vi "Prober_ProbeTouchdown.vi"(8 "error in (no error)":errorcluster, 11 "AlessiRel6100 in":refnum<class "AlessiRel6100.lvclass">) -> (0 "error out":errorcluster, 1 "previous Z [µm]":i32, 2 "Z [µm]":i32, 3 "AlessiRel6100 out":refnum<class "AlessiRel6100.lvclass">)   [LabVIEW 2018, in "AlessiRel6100.lvclass"]
uses:
  AlessiRel6100.lvclass
  InstrumentSetup.vi
  <vilib>/Utility/error.llb/Error Cluster From Error Code.vi
  <vilib>/ErrorRing/Error Ring.xnode
  ArduinoControl/ArduinoControl.lvclass
  InstrControl.lvclass
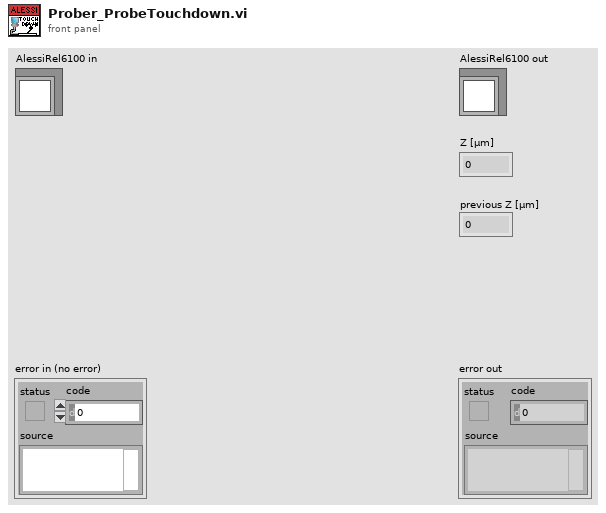
[diagram p1: front panel]
types:
  T1 = cluster{"touchdown height [µm]":i32, "search band [µm]":u32, "speed [µm/step]":u32, "overdrive [µm]":u32}
  T2 = cluster{"VISA address":refnum<visa-resource-name>, "T sensor":enum16{"SHT", "DS"}, "Arduino":refnum<class "ArduinoControl.lvclass">}
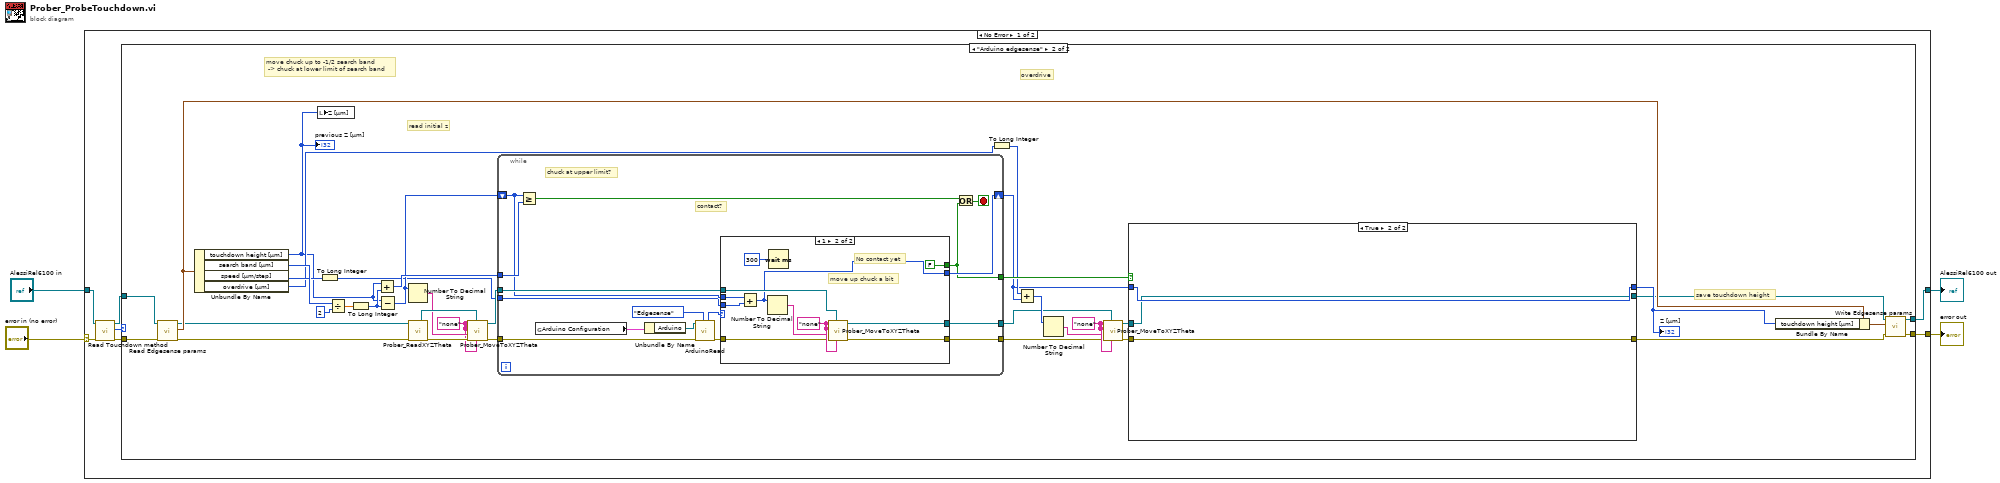
[diagram p0: block diagram]
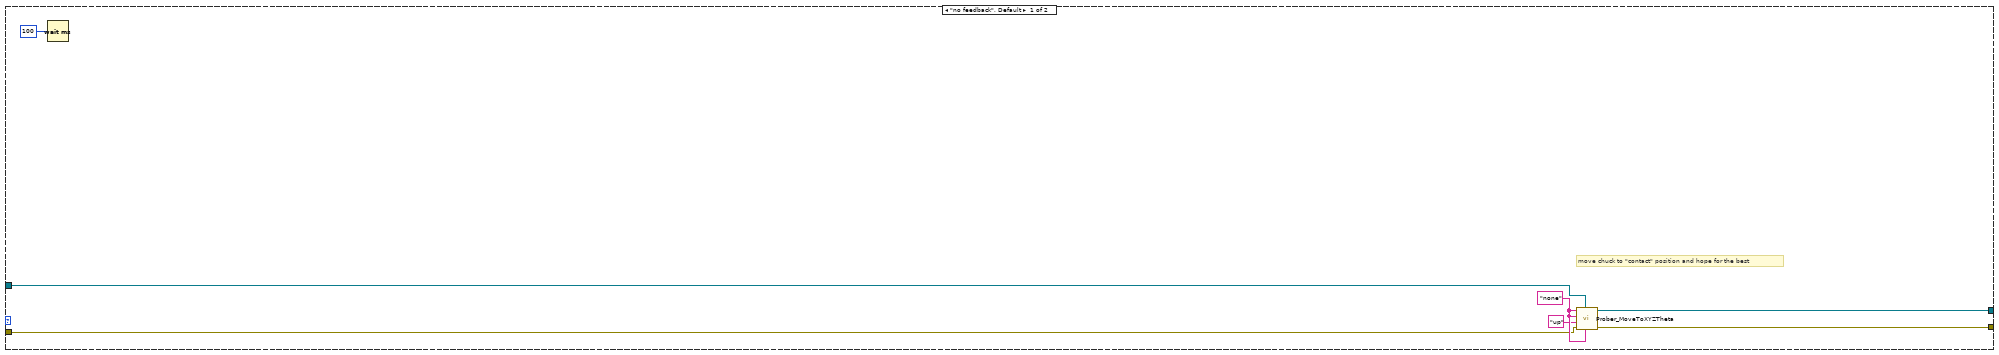
[diagram p2: hidden frame]
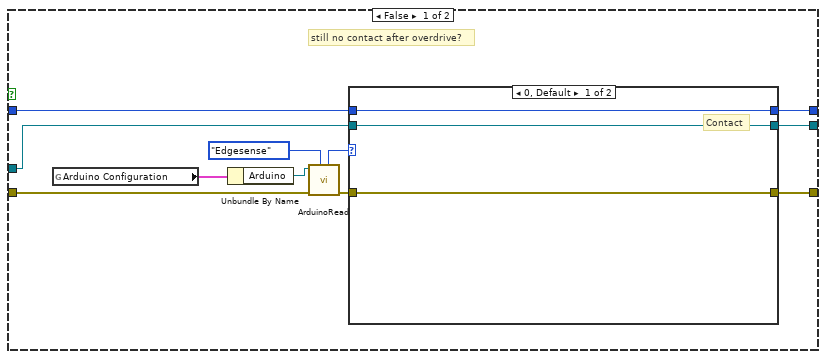
[diagram p3: hidden frame]
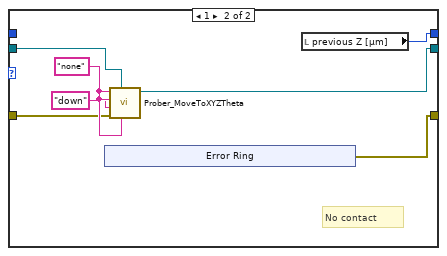
[diagram p4: hidden frame]
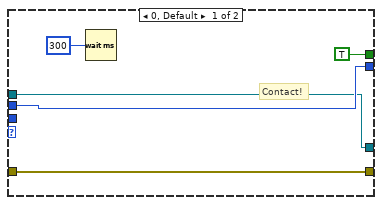
[diagram p5: hidden frame]
diagram:
  n1 = case shown="No Error" "error in (no error)" {
    selector: "error in (no error)" -> [w8 w118]
    tunnel: [w11 w118] -> w1
    tunnel: [w10 w117] -> w2
    tunnel: "AlessiRel6100 in" -> [w9 w117]
    frame No Error {
      n2 = call-dynamic "Read Touchdown method.vi"("error in (no error)"=w8, "AlessiRel6100 in"=w9) -> ("error out"=w6:errorcluster, "Touchdown method"=w7:enum16{"no feedback", "Arduino edgesense"}, "AlessiRel6100 out"=w5:refnum<class "AlessiRel6100.lvclass">)  [unwired: 7 in]
      n3 = case shown="\"Arduino edgesense\"" w7 {
        tunnel: w5 -> [w15 w28]
        tunnel: w6 -> [w14 w27]
        tunnel: [w12 w19] -> w11
        tunnel: [w13 w20] -> w10
        frame "no feedback", Default {
          w17 = "none"
          # "move chuck to \"contact\" position and hope for the best"
          n4 = Wait (ms)(milliseconds to wait=100) -> ()  [unwired: 1 out]
          n5 = call-dynamic "Prober_MoveToXYZTheta.vi"("Theta location [mdeg]"=w17, "AlessiRel6100 in"=w15, "error in (no error)"=w14, "Z location [µm]"="up", "Y location [µm]"=w17, "X location [µm]"=w17) -> ("error out"=w12:errorcluster, "AlessiRel6100 out"=w13:refnum<class "AlessiRel6100.lvclass">)  [unwired: 3 in, 1 out]
        }
        frame "Arduino edgesense" {
          w40 = "none" ("Z location")
          w46 = "none" ("Z location")
          # "save touchdown height"
          # "overdrive"
          # "read initial z"
          # "move chuck up to -1/2 search band\n -> chuck at lower limit of search band"
          n6 = call-dynamic "Read Edgesense params.vi"("error in (no error)"=w27, "AlessiRel6100 in"=w28) -> ("error out"=w24:errorcluster, "Edgesense params"=w26:T1, "AlessiRel6100 out"=w25:refnum<class "AlessiRel6100.lvclass">)  [unwired: 7 in]
          n7 = Unbundle By Name(w26) -> ("touchdown height [µm]"=w29:i32, "search band [µm]"=w51:u32, "speed [µm/step]"=w43:u32, "overdrive [µm]"=w33:u32)
          "previous Z [µm]" <- w29
          n8 = local write "Z [µm]"(w29) -> ()
          n9 = To Long Integer(number=w43) -> (32bit integer=w42:i32)
          n10 = Divide(x=w51, y=u32 2) -> (x/y=w50:dbl)
          n11 = To Long Integer(number=w50) -> (32bit integer=w49:i32)
          n12 = Add(x=w29, y=w49) -> (x+y=w48:i32)
          n13 = Subtract(x=w29, y=w49) -> (x-y=w44:i32)
          n14 = Number To Decimal String(number=w44) -> (decimal integer string=w52:string)  [unwired: 1 in]
          n15 = call-dynamic "Prober_ReadXYZTheta.vi"("error in (no error)"=w24, "AlessiRel6100 in"=w25) -> ("error out"=w54:errorcluster, "AlessiRel6100 out"=w53:refnum<class "AlessiRel6100.lvclass">)  [unwired: 4 in, 4 out]
          n16 = call-dynamic "Prober_MoveToXYZTheta.vi"("Theta location [mdeg]"=w46, "AlessiRel6100 in"=w53, "error in (no error)"=w54, "Z location [µm]"=w52, "Y location [µm]"=w46, "X location [µm]"=w46) -> ("error out"=w47:errorcluster, "AlessiRel6100 out"=w45:refnum<class "AlessiRel6100.lvclass">)  [unwired: 3 in, 1 out]
          n17 = while {
            tunnel: w48 -> [w100]
            shift-right: [w87] -> w31
            shift-left: w44 -> [w88]
            tunnel: w47 -> [w98]
            tunnel: w42 -> [w86]
            tunnel: w45 -> [w91]
            tunnel: [w90] -> w36
            tunnel: [w89] -> w37
            tunnel: [w85] -> w41
            stop <- w94 stop-if-true
            # "contact?"
            # "chuck at upper limit?"
            n18 = Greater Or Equal?(x=w88, y=w100) -> (x >= y?=w93:bool)
            n19 = global read "InstrumentSetup.vi" "Arduino Configuration"() -> (w97:T2)
            n20 = Unbundle By Name(w97) -> ("Arduino"=w96:refnum<class "ArduinoControl.lvclass">)
            n21 = call "ArduinoRead.vi"("Arduino function"=enum16{"T/RH", "Interlock", "Edgesense"}."Edgesense", "error in (no error)"=w98, "ArduinoControl in"=w96) -> ("error out"=w92:errorcluster, "Edgesense Status"=w95:u16)  [unwired: 3 in, 4 out]
            n22 = case shown="1" w95 {
              tunnel: w86 -> [_ w116]
              tunnel: w88 -> [w102 w107]
              tunnel: [w102 w106] -> w87
              tunnel: [TRUE FALSE] -> w85
              tunnel: w92 -> [w104 w112]
              tunnel: [w104 w111] -> w89
              tunnel: w91 -> [w101 w109]
              tunnel: [w101 w108] -> w90
              frame 0, Default {
                # "Contact!"
                n23 = Wait (ms)(milliseconds to wait=300) -> ()  [unwired: 1 out]
              }
              frame 1 {
                w114 = "none" ("Z location")
                # "No contact yet"
                # "move up chuck a bit"
                n24 = Add(x=w107, y=w116) -> (x+y=w106:i32)
                n25 = Number To Decimal String(number=w106) -> (decimal integer string=w113:string)  [unwired: 1 in]
                n26 = Wait (ms)(milliseconds to wait=300) -> ()  [unwired: 1 out]
                n27 = call-dynamic "Prober_MoveToXYZTheta.vi"("Theta location [mdeg]"=w114, "AlessiRel6100 in"=w109, "error in (no error)"=w112, "Z location [µm]"=w113, "Y location [µm]"=w114, "X location [µm]"=w114) -> ("error out"=w111:errorcluster, "AlessiRel6100 out"=w108:refnum<class "AlessiRel6100.lvclass">)  [unwired: 3 in, 1 out]
              }
            }
            n28 = Or(x=w93, y=w85) -> (x .or. y?=w94:bool)
          }
          n29 = To Long Integer(number=w33) -> (32bit integer=w32:i32)
          n30 = Add(x=w32, y=w31) -> (x+y=w39:i32)
          n31 = Number To Decimal String(number=w39) -> (decimal integer string=w38:string)  [unwired: 1 in]
          n32 = call-dynamic "Prober_MoveToXYZTheta.vi"("Theta location [mdeg]"=w40, "AlessiRel6100 in"=w36, "error in (no error)"=w37, "Z location [µm]"=w38, "Y location [µm]"=w40, "X location [µm]"=w40) -> ("error out"=w35:errorcluster, "AlessiRel6100 out"=w34:refnum<class "AlessiRel6100.lvclass">)  [unwired: 3 in, 1 out]
          n33 = case shown="True" w41 {
            tunnel: w35 -> [w63 w82]
            tunnel: w34 -> [w61 w83]
            tunnel: w31 -> [w59 w84]
            tunnel: [w58 w84] -> w30
            tunnel: [w57 w83] -> w21
            tunnel: [w56 w82] -> w23
            frame False {
              # "still no contact after overdrive?"
              n34 = global read "InstrumentSetup.vi" "Arduino Configuration"() -> (w65:T2)
              n35 = Unbundle By Name(w65) -> ("Arduino"=w66:refnum<class "ArduinoControl.lvclass">)
              n36 = call "ArduinoRead.vi"("Arduino function"=enum16{"T/RH", "Interlock", "Edgesense"}."Edgesense", "error in (no error)"=w63, "ArduinoControl in"=w66) -> ("error out"=w60:errorcluster, "Edgesense Status"=w62:u16)  [unwired: 3 in, 4 out]
              n37 = case shown="0, Default" w62 {
                tunnel: w61 -> [w68 w73]
                tunnel: w60 -> [w67 w72]
                tunnel: w59 -> [w69 _]
                tunnel: [w69 w76] -> w58
                tunnel: [w68 w71] -> w57
                tunnel: [w67 w70] -> w56
                frame 0, Default {
                  # "Contact"
                }
                frame 1 {
                  w75 = "none" ("Z location")
                  # "No contact"
                  n38 = xnode "Error Ring"() -> ("error out"=w70:errorcluster)
                  n39 = call-dynamic "Prober_MoveToXYZTheta.vi"("Theta location [mdeg]"=w75, "AlessiRel6100 in"=w73, "error in (no error)"=w72, "Z location [µm]"="down", "Y location [µm]"=w75, "X location [µm]"=w75) -> ("AlessiRel6100 out"=w71:refnum<class "AlessiRel6100.lvclass">)  [unwired: 3 in, 2 out]
                  n40 = local read "previous Z [µm]"() -> (w76:i32)
                }
              }
            }
            frame True {
            }
          }
          "Z [µm]" <- w30
          n41 = Bundle By Name(cluster=w26, "touchdown height [µm]"=w30) -> (w22:T1)
          n42 = call-dynamic "Write Edgesense params.vi"("error in (no error)"=w23, "Edgesense params"=w22, "AlessiRel6100 in"=w21) -> ("error out"=w19:errorcluster, "AlessiRel6100 out"=w20:refnum<class "AlessiRel6100.lvclass">)  [unwired: 7 in]
        }
      }
    }
    frame Error {
    }
  }
  "error out" <- w1
  "AlessiRel6100 out" <- w2
